vi "RequestSweepReport.vi"(8 "UiDefinition 2":T1) -> ()   [LabVIEW 2020]
uses:
  UIReferences.ctl
  D:/LabviewDXFViewer/LabviewDXFViewer/bin/Release/LabviewDXFViewer.exe
  LabviewDXFViewer/bin/Release/LabviewDXFViewer.exe
  <vilib>/httpClient/LabVIEWHTTPClient.lvlib
panel:
  out "error out":errorcluster
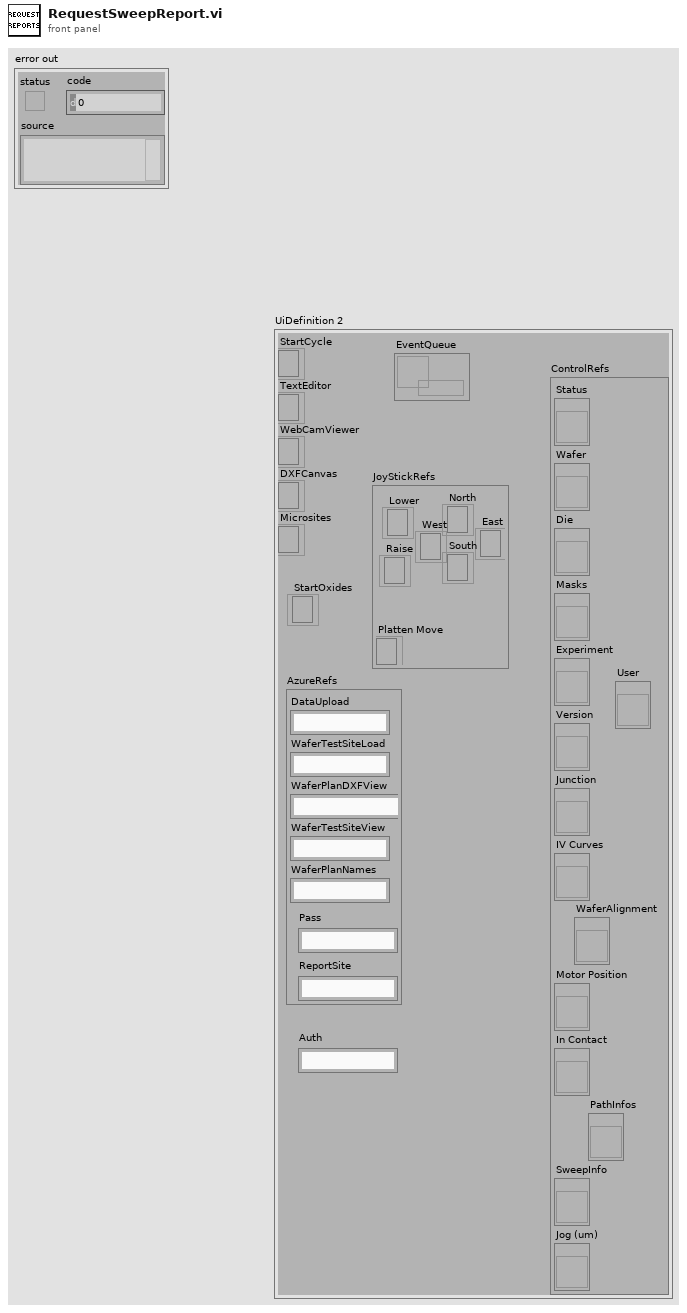
[diagram p1: front panel]
types:
  T1 = typedef "UIReferences.ctl" = cluster{"StartCycle":refnum<k24>, "TextEditor":refnum<k24>, "WebCamViewer":refnum<k24>, "DXFCanvas":refnum<k24>, "Microsites":refnum<k24>, "JoyStickRefs":cluster{"North":refnum<k24>, "Lower":refnum<k24>, "Raise":refnum<k24>, "Platten Move":refnum<k24>, "West":refnum<k24>, "East":refnum<k24>, "South":refnum<k24>}, "AzureRefs":cluster{"DataUpload":string, "WaferTestSiteLoad":string, "WaferPlanDXFView":string, "WaferTestSiteView":string, "WaferPlanNames":string, "Pass":string, "ReportSite":string}, "ControlRefs":cluster{"Status":refnum<vi>, "Wafer":refnum<vi>, "Die":refnum<vi>, "Masks":refnum<vi>, "Experiment":refnum<vi>, "Version":refnum<vi>, "Junction":refnum<vi>, "IV Curves":refnum<vi>, "Motor Position":refnum<vi>, "In Contact":refnum<vi>, "SweepInfo":refnum<vi>, "Jog (um)":refnum<vi>, "PathInfos":refnum<vi>, "User":refnum<vi>, "WaferAlignment":refnum<vi>}, "EventQueue":refnum<queue>, "StartOxides":refnum<k24>, "Auth":string}
  T2 = typedef "LabVIEWHTTPClient.lvlib/ClientHandle.ctl" = refnum<k1>
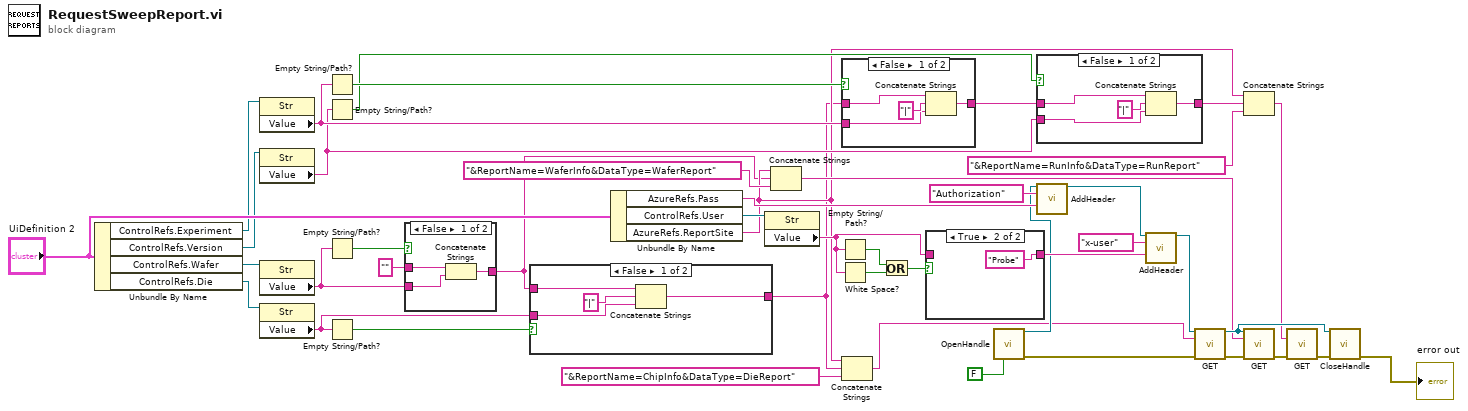
[diagram p0: block diagram]
diagram:
  n1 = Unbundle By Name("UiDefinition 2") -> ("ControlRefs.Experiment"=w19:refnum<vi>, "ControlRefs.Version"=w16:refnum<vi>, "ControlRefs.Wafer"=w28:refnum<vi>, "ControlRefs.Die"=w23:refnum<vi>)
  n2 = property class="Str"(reference=w19) -> ("Value"=w20:string)  [unwired: 1 in, 2 out]
  n3 = property class="Str"(reference=w16) -> ("Value"=w17:string)  [unwired: 1 in, 2 out]
  n4 = property class="Str"(reference=w28) -> ("Value"=w25:string)  [unwired: 1 in, 2 out]
  n5 = property class="Str"(reference=w23) -> ("Value"=w22:string)  [unwired: 1 in, 2 out]
  n6 = Empty String/Path?(string/path=w20) -> (empty?=w21:bool)
  n7 = Empty String/Path?(string/path=w17) -> (empty?=w18:bool)
  n8 = Empty String/Path?(string/path=w25) -> (empty?=w26:bool)
  n9 = Empty String/Path?(string/path=w22) -> (empty?=w24:bool)
  n10 = case shown="False" w26 {
    tunnel: "" -> [w47 w48]
    tunnel: [w46 w48] -> w2
    tunnel: w25 -> [w45 _]
    frame False {
      n11 = Concatenate Strings(w47, w45) -> (w46:string)
    }
    frame True {
    }
  }
  n12 = case shown="False" w24 {
    tunnel: w2 -> [w52 w53]
    tunnel: [w51 w53] -> w1
    tunnel: w22 -> [w49 _]
    frame False {
      n13 = Concatenate Strings(w52, "|" ("string"), w49) -> (w51:string)
    }
    frame True {
    }
  }
  n14 = Unbundle By Name("UiDefinition 2") -> ("AzureRefs.Pass"=w40:string, "ControlRefs.User"=w38:refnum<vi>, "AzureRefs.ReportSite"=w6:string)
  n15 = property class="Str"(reference=w38) -> ("Value"=w33:string)  [unwired: 1 in, 2 out]
  n16 = Concatenate Strings(w6, w2, "&ReportName=WaferInfo&DataType=WaferReport" ("string")) -> (w9:string)
  n17 = Empty String/Path?(string/path=w33) -> (empty?=w34:bool)
  n18 = White Space?(1:w33) -> (0:w37:bool)
  n19 = case shown="False" w21 {
    tunnel: w1 -> [w57 w58]
    tunnel: [w56 w58] -> w15
    tunnel: w20 -> [w54 _]
    frame False {
      n20 = Concatenate Strings(w57, "|" ("string"), w54) -> (w56:string)
    }
    frame True {
    }
  }
  n21 = Concatenate Strings(w6, w1, "&ReportName=ChipInfo&DataType=DieReport" ("string")) -> (w30:string)
  n22 = Or(x=w34, y=w37) -> (x .or. y?=w35:bool)
  n23 = case shown="True" w35 {
    tunnel: w33 -> [w59 _]
    tunnel: [w59 "Probe"] -> w36
    frame False {
    }
    frame True {
    }
  }
  n24 = call <vilib>:"OpenHandle.vi"("verify server(true)"=FALSE) -> ("client handle out"=w32:T2, "error out"=w43:errorcluster)  [unwired: 13 in]
  n25 = case shown="False" w18 {
    tunnel: w15 -> [w64 w65]
    tunnel: [w63 w65] -> w5
    tunnel: w17 -> [w61 _]
    frame False {
      n26 = Concatenate Strings(w64, "|" ("string"), w61) -> (w63:string)
    }
    frame True {
    }
  }
  n27 = call <vilib>:"AddHeader.vi"("client handle"=w32, "header"="Authorization", "value"=w40) -> ("client handle out"=w42:T2)  [unwired: 11 in, 1 out]
  n28 = call <vilib>:"AddHeader.vi"("client handle"=w42, "header"="x-user", "value"=w36) -> ("client handle out"=w13:T2)  [unwired: 11 in, 1 out]
  n29 = call <vilib>:"GET.vi"("client handle"=w13, "url"=w30, "error in (no error)"=w43) -> ("client handle out"=w10:T2, "error out"=w11:errorcluster)  [unwired: 9 in, 2 out]
  n30 = Concatenate Strings(w6, w5, "&ReportName=RunInfo&DataType=RunReport" ("string")) -> (w7:string)
  n31 = call <vilib>:"GET.vi"("client handle"=w10, "url"=w9, "error in (no error)"=w11) -> ("error out"=w4:errorcluster)  [unwired: 9 in, 3 out]
  n32 = call <vilib>:"GET.vi"("url"=w7, "error in (no error)"=w4) -> ("error out"=w3:errorcluster)  [unwired: 10 in, 3 out]
  n33 = call <vilib>:"CloseHandle.vi"("client handle"=w10, "error in (no error)"=w3) -> ("error out"=→"error out":errorcluster)  [unwired: 13 in]
